vi "DigitalOutput Reservations.vi"(4 "Reset":bool, 6 "Timestamp line":tag, 7 "Line":tag) -> (0 "Exit code":T1, 1 "Index assigned":i32, 2 "DO timestamp lines":tag[](array[tag]), 3 "DigitalOutput lines":tag[](array[tag]))   [LabVIEW 2015]
doc: "Attempt to reserve a line as a digital output, with a cooresponding timestamp line. This also returns a list of lines that have been previously reserved.\n\nAs a Device developer, just call this with the line you want to add, check that the exit code is good, and save the assigned index.\n\nAs a Rack developer, remember to reset the reservations list before Device initialization and then call it with an empty line afterwards to get the list of digital output lines."
uses:
  Typedefs/Reservation exit codes.ctl
  <vilib>/Utility/error.llb/DialogType.ctl
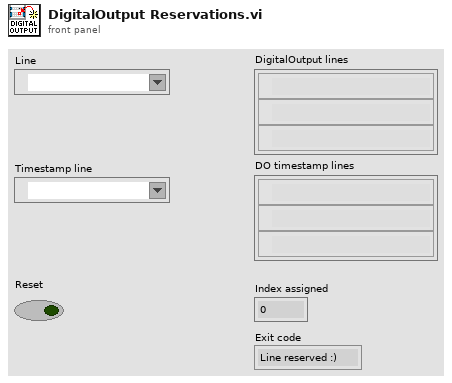
[diagram p1: front panel]
types:
  T1 = typedef "Reservation exit codes.ctl" = enum16{"Line reserved :)", "List reset.", "Empty line!", "Bad line!", "Already reserved!", "Timestamp conflict!", "Timestamp empty."}
  T2 = typedef "DialogType.ctl" = u16
  T3 = enum16{"Analog input", "Analog output", "Digital input", "Digital output", "Counter input", "Counter output"}
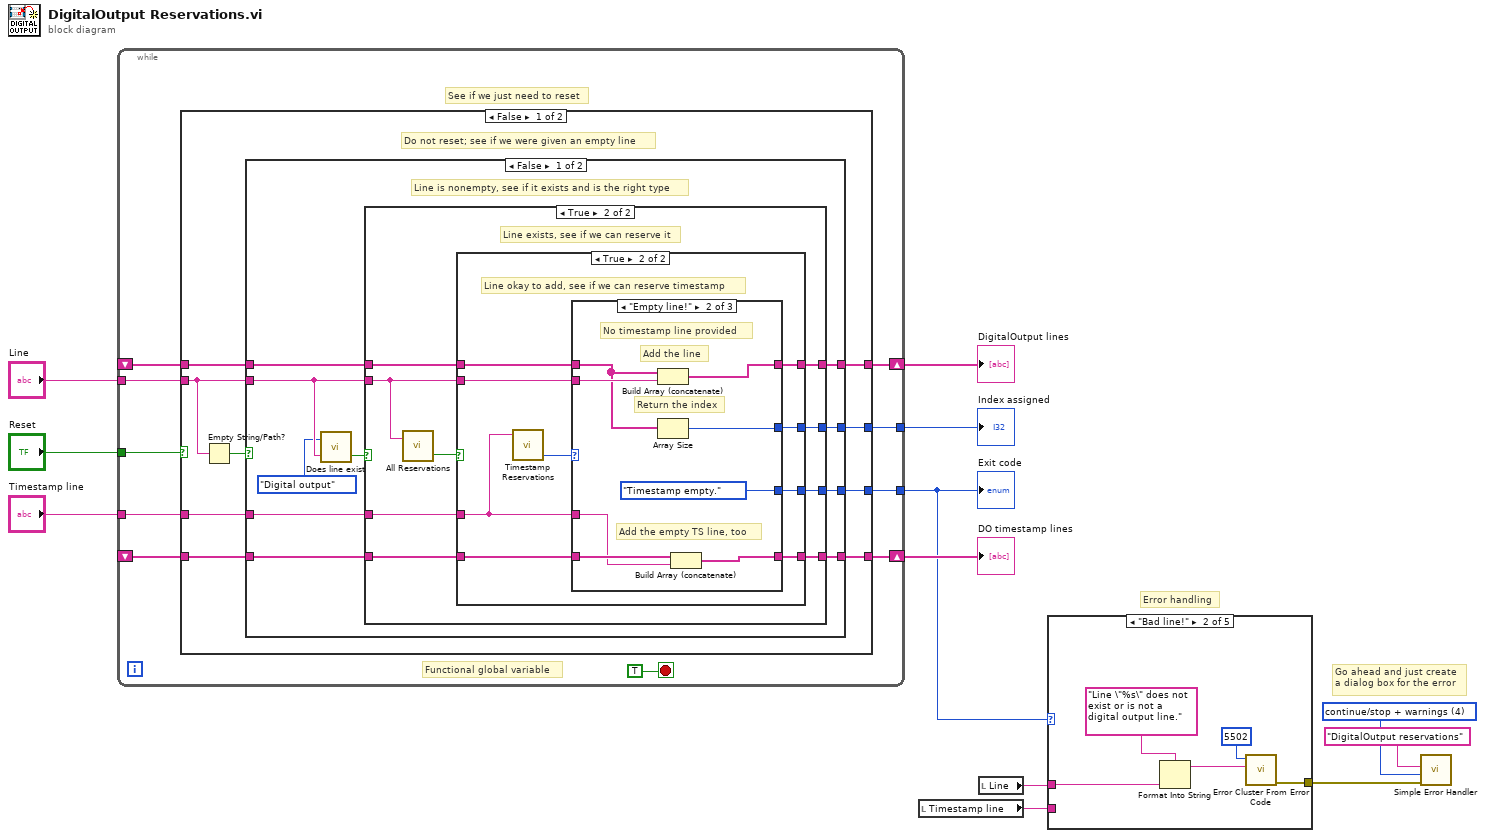
[diagram p0: block diagram]
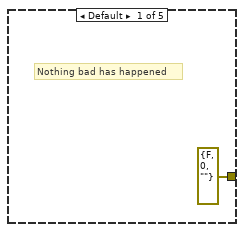
[diagram p2: hidden frame]
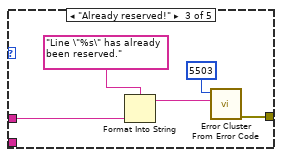
[diagram p3: hidden frame]
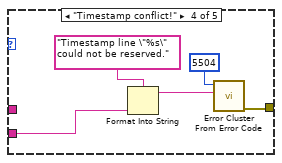
[diagram p4: hidden frame]
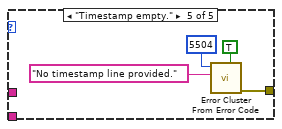
[diagram p5: hidden frame]
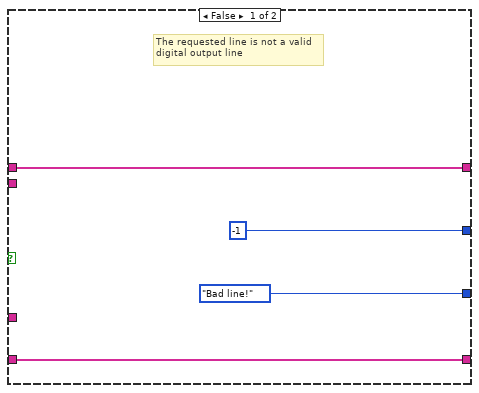
[diagram p6: hidden frame]
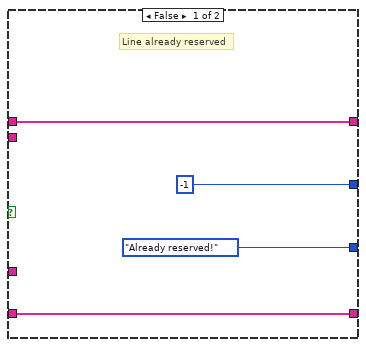
[diagram p7: hidden frame]
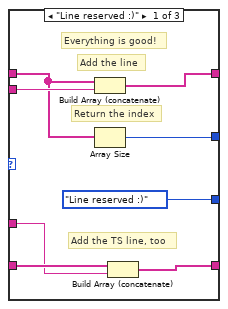
[diagram p8: hidden frame]
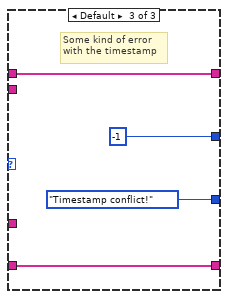
[diagram p9: hidden frame]
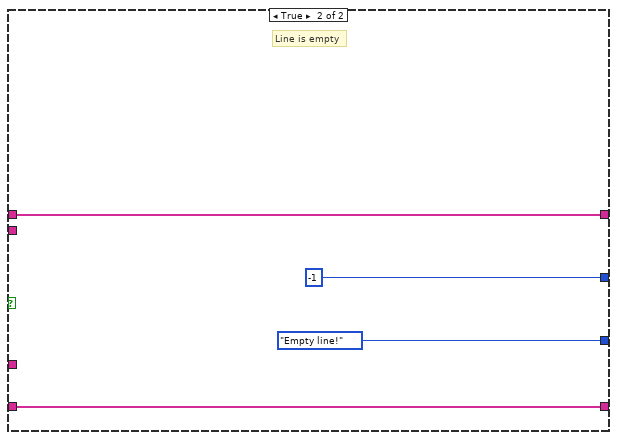
[diagram p10: hidden frame]
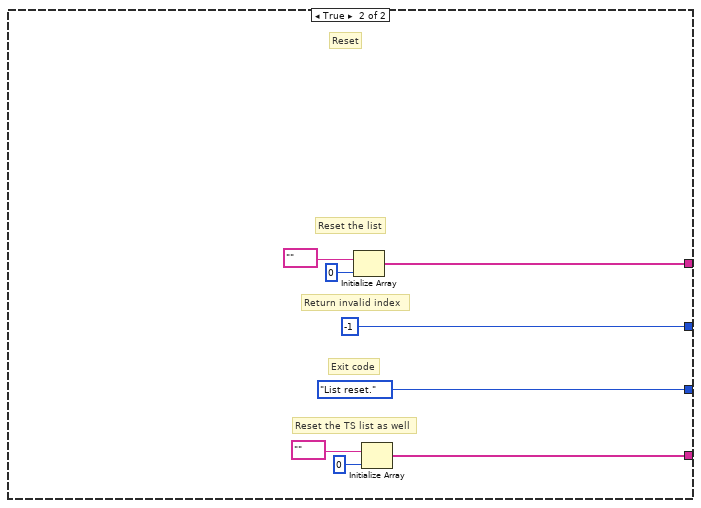
[diagram p11: hidden frame]
diagram:
  w5 = T2 4 items=["no dialog", "OK message", "continue or stop message", "OK message + warnings", "continue/stop + warnings"] ("type of dialog (OK msg:1)")
  # "Error handling"
  # "Go ahead and just create\na dialog box for the error"
  n1 = while {
    tunnel: [w22] -> w3
    tunnel: "Reset" -> [w21]
    shift-right: [w20] -> w12
    shift-left: _ -> [w18]
    tunnel: "Line" -> [w17]
    tunnel: [w16] -> w10
    tunnel: "Timestamp line" -> [w15]
    shift-right: [w13] -> w7
    shift-left: _ -> [w14]
    stop <- TRUE ("stop") stop-if-true
    # "See if we just need to reset"
    # "Functional global variable"
    n2 = case shown="False" w21 {
      tunnel: [w28 Reservation_exit_codes."List reset." ("Exit code")] -> w22
      tunnel: [w31 w98] -> w20
      tunnel: w18 -> [w30 _]
      tunnel: w17 -> [w26 _]
      tunnel: [w29 -1 ("Index assigned")] -> w16
      tunnel: w15 -> [w25 _]
      tunnel: [w24 w92] -> w13
      tunnel: w14 -> [w23 _]
      frame False {
        # "Do not reset; see if we were given an empty line"
        n3 = Empty String/Path?(string/path=w26) -> (empty?=w27:bool)
        n4 = case shown="False" w27 {
          tunnel: [w41 w91] -> w31
          tunnel: w30 -> [w40 w91]
          tunnel: [w39 -1] -> w29
          tunnel: [w38 Reservation_exit_codes."Empty line!" ("Exit code")] -> w28
          tunnel: w26 -> [w36 _]
          tunnel: w25 -> [w34 _]
          tunnel: [w33 w88] -> w24
          tunnel: w23 -> [w32 w88]
          frame False {
            # "Line is nonempty, see if it exists and is the right type"
            n5 = call "Does line exist.vi"("Line to look for"=w36, "Line type"=T3."Digital output") -> ("Does line exist?"=w37:bool)  [unwired: 1 out]
            n6 = case shown="True" w37 {
              tunnel: [w45 w54] -> w41
              tunnel: w40 -> [w45 w53]
              tunnel: [-1 w52] -> w39
              tunnel: [Reservation_exit_codes."Bad line!" ("Exit code") w51] -> w38
              tunnel: w36 -> [_ w49]
              tunnel: w34 -> [_ w48]
              tunnel: [w42 w47] -> w33
              tunnel: w32 -> [w42 w46]
              frame False {
                # "The requested line is not a valid\ndigital output line"
              }
              frame True {
                # "Line exists, see if we can reserve it"
                n7 = call "All Reservations.vi"("Line to add"=w49) -> ("Line added?"=w50:bool)  [unwired: 1 in, 1 out]
                n8 = case shown="True" w50 {
                  tunnel: w53 -> [w58 w65]
                  tunnel: [w58 w67] -> w54
                  tunnel: w49 -> [_ w66]
                  tunnel: [-1 w64] -> w52
                  tunnel: [Reservation_exit_codes."Already reserved!" ("Exit code") w63] -> w51
                  tunnel: w48 -> [_ w62]
                  tunnel: [w55 w61] -> w47
                  tunnel: w46 -> [w55 w60]
                  frame False {
                    # "Line already reserved"
                  }
                  frame True {
                    # "Line okay to add, see if we can reserve timestamp"
                    n9 = call "Timestamp Reservations.vi"("Line"=w62) -> ("Exit code"=w59:T1)  [unwired: 2 in, 2 out]
                    n10 = case shown="\"Empty line!\"" w59 {
                      tunnel: [w75 w83 w87] -> w67
                      tunnel: w66 -> [w74 w82 _]
                      tunnel: w65 -> [w73 w81 w87]
                      tunnel: [w72 w80 -1] -> w64
                      tunnel: [Reservation_exit_codes."Line reserved :)" ("Exit code") Reservation_exit_codes."Timestamp empty." ("Exit code") Reservation_exit_codes."Timestamp conflict!" ("Exit code")] -> w63
                      tunnel: w62 -> [w68 w76 _]
                      tunnel: [w70 w78 w84] -> w61
                      tunnel: w60 -> [w69 w77 w84]
                      frame "Line reserved :)" {
                        # "Add the TS line, too"
                        # "Everything is good!"
                        # "Return the index"
                        # "Add the line"
                        n11 = Build Array (concatenate)(w73, w74) -> (w75:tag[])
                        n12 = Array Size(array=w73) -> (size(s)=w72:i32)
                        n13 = Build Array (concatenate)(w69, w68) -> (w70:tag[])
                      }
                      frame "Empty line!" {
                        # "Add the empty TS line, too"
                        # "No timestamp line provided"
                        # "Return the index"
                        # "Add the line"
                        n14 = Build Array (concatenate)(w81, w82) -> (w83:tag[])
                        n15 = Array Size(array=w81) -> (size(s)=w80:i32)
                        n16 = Build Array (concatenate)(w77, w76) -> (w78:tag[])
                      }
                      frame Default {
                        # "Some kind of error\nwith the timestamp"
                      }
                    }
                  }
                }
              }
            }
          }
          frame True {
            # "Line is empty"
          }
        }
      }
      frame True {
        # "Reset the TS list as well"
        # "Reset"
        # "Exit code"
        # "Return invalid index"
        # "Reset the list"
        n17 = Initialize Array(tag "" ("Line to add"), 0 ("dimension size")) -> (w98:tag[])
        n18 = Initialize Array(tag "" ("Line to add"), 0 ("dimension size")) -> (w92:tag[])
      }
    }
  }
  "DigitalOutput lines" <- w12
  "Exit code" <- w3
  "Index assigned" <- w10
  "DO timestamp lines" <- w7
  n19 = local read "Timestamp line"() -> (w1:tag)
  n20 = local read "Line"() -> (w2:tag)
  n21 = case shown="\"Bad line!\"" w3 {
    tunnel: w2 -> [_ w102 w106 _ _]
    tunnel: [errorcluster {"status"=FALSE, "code"=0, "source"=""} ("error out") w101 w107 w112 w118] -> w4
    tunnel: w1 -> [_ _ _ w111 _]
    frame Default {
      # "Nothing bad has happened"
    }
    frame "Bad line!" {
      n22 = Format Into String(format string="Line \"%s\" does not exist or is not a digital output line.", w102) -> (resulting string=w105:string)  [unwired: 2 in, 1 out]
      n23 = call <vilib>:"Error Cluster From Error Code.vi"("error message (\"\")"=w105, "error code (0)"=5502) -> ("error out"=w101:errorcluster)  [unwired: 7 in]
    }
    frame "Already reserved!" {
      n24 = Format Into String(format string="Line \"%s\" has already been reserved.", w106) -> (resulting string=w108:string)  [unwired: 2 in, 1 out]
      n25 = call <vilib>:"Error Cluster From Error Code.vi"("error message (\"\")"=w108, "error code (0)"=5503) -> ("error out"=w107:errorcluster)  [unwired: 7 in]
    }
    frame "Timestamp conflict!" {
      n26 = Format Into String(format string="Timestamp line \"%s\" could not be reserved.", w111) -> (resulting string=w113:string)  [unwired: 2 in, 1 out]
      n27 = call <vilib>:"Error Cluster From Error Code.vi"("error message (\"\")"=w113, "error code (0)"=5504) -> ("error out"=w112:errorcluster)  [unwired: 7 in]
    }
    frame "Timestamp empty." {
      n28 = call <vilib>:"Error Cluster From Error Code.vi"("is warning? (False)"=TRUE, "error message (\"\")"="No timestamp line provided." ("error message (\"\")"), "error code (0)"=5504) -> ("error out"=w118:errorcluster)  [unwired: 6 in]
    }
  }
  n29 = call <vilib>:"Simple Error Handler.vi"("error source (\" \")"="DigitalOutput reservations" ("error source (\" \")"), "type of dialog (OK msg:1)"=w5, "error in (no error)"=w4) -> ()  [unwired: 2 in, 5 out]
